vi "Flush.vi"(8 "error in":errorcluster, 11 "Message Buffer in":refnum<class "Message Buffer.lvclass">) -> (0 "error out":errorcluster, 2 "Messages":refnum<class "IMessage.lvclass">[](array[class]), 3 "Message Buffer out":refnum<class "Message Buffer.lvclass">)   [LabVIEW 2024, in "PCAN.lvlib" / "Message Buffer.lvclass"]
uses:
  Message Buffer.lvclass
  Interfaces/IMessage/IMessage.lvclass
  Message Buffer.lvclass/Message Buffer.ctl
  CAN Message/CAN Message.lvclass
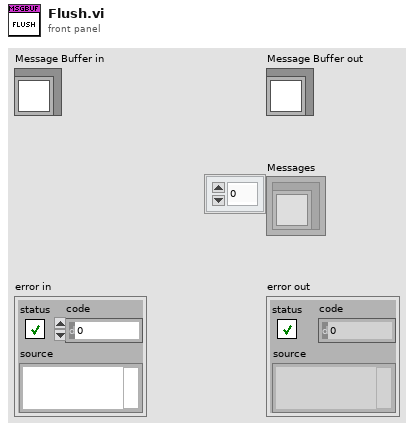
[diagram p1: front panel]
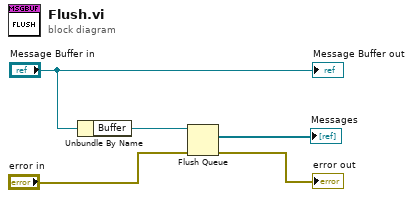
[diagram p0: block diagram]
diagram:
  n1 = Unbundle By Name("Message Buffer in") -> ("Buffer"=w1:refnum<queue>)
  n2 = Flush Queue(queue=w1, error in (no error)="error in") -> (remaining elements=→"Messages":refnum<class "CAN Message.lvclass">[], error out=→"error out":errorcluster)  [unwired: 1 out]
  "Message Buffer out" <- "Message Buffer in"
